vi "Run.vi"(8 "error in (no error)":errorcluster, 10 "Control In":T1={"I-O.lvclass"=refnum, "Gantry"=refnum, "Dispenser"="COM1"}, 11 "Assembly In":refnum<class "Assembly Run.lvclass">) -> (0 "error out":errorcluster, 2 "Control Out":T1={"I-O.lvclass"=refnum, "Gantry"=refnum, "Dispenser"="COM1"}, 3 "Assembly Out":refnum<class "Assembly Run.lvclass">)   [LabVIEW 2018, in "Assembly Run.lvclass"]
uses:
  Assembly Run.lvclass
  Controller/Controllers.ctl
  Controller/I-O/I-O.lvclass
  C:/Program Files (x86)/Aerotech/A3200/LabVIEW/2010/Bin/Aerotech.A3200.dll
  Program Files (x86)/Aerotech/A3200/LabVIEW/2010/Bin/Aerotech.A3200.dll
  Assembly Run.lvclass/Assembly Run.ctl
  Workspace/Fixture.lvclass
  Routine/Routine.lvclass
  Controller/Motion/Motion.lvclass
  Controller/Controller.lvclass
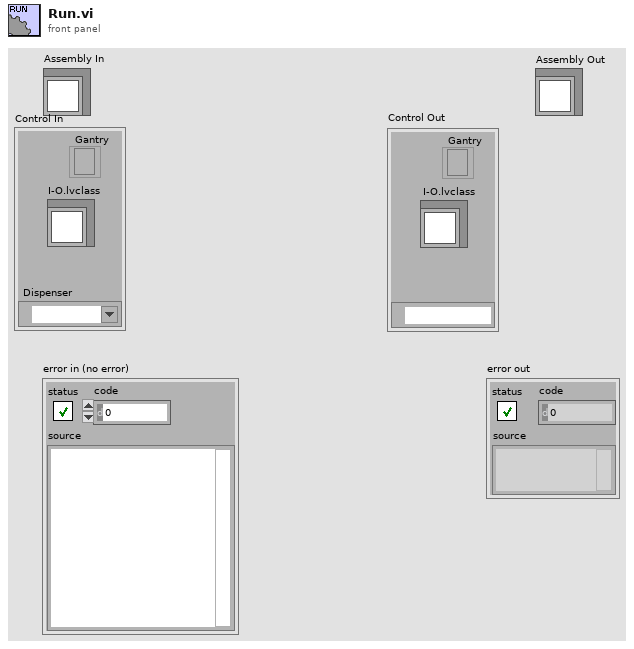
[diagram p1: front panel]
types:
  T1 = typedef "Controller.lvclass/Controllers.ctl" = cluster{"I-O.lvclass":refnum<class "I-O.lvclass">, "Gantry":refnum<k24>, "Dispenser":refnum<visa-resource-name>}
  T2 = typedef "Fixture.lvclass/Workspace.ctl" = cluster{"XYZTheta":dbl[], "Workspace Valve":i32, "Workspace Sensor":i32}
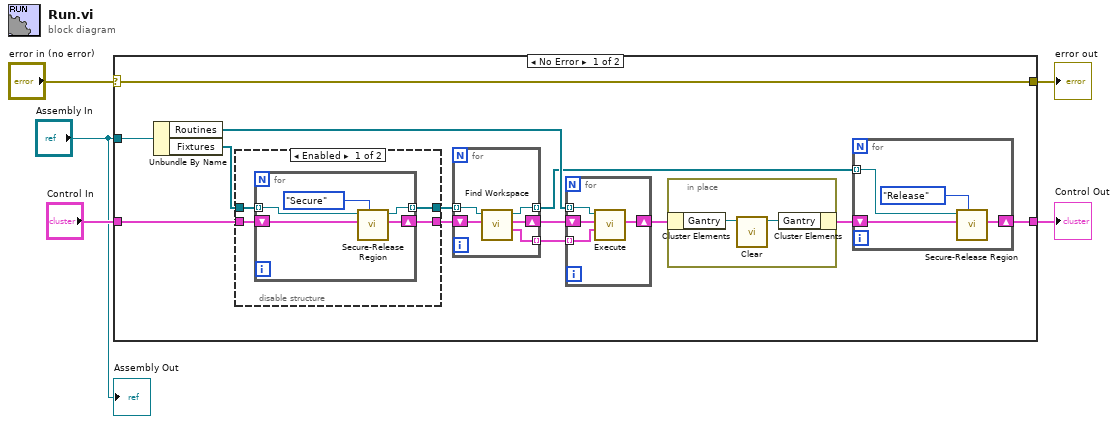
[diagram p0: block diagram]
diagram:
  n1 = case shown="No Error" "error in (no error)" {
    selector: "error in (no error)" -> [w18 w46]
    tunnel: [w18 w46] -> w4
    tunnel: [w12 w45] -> w3
    tunnel: "Assembly In" -> [w10 _]
    tunnel: "Control In" -> [w7 w45]
    frame No Error {
      n2 = Unbundle By Name(w10) -> ("Routines"=w17:refnum<class "Routine.lvclass">[], "Fixtures"=w11:refnum<class "Fixture.lvclass">[])
      n3 = disable-structure shown="Enabled" {
        disable-tunnel: [w22 w29] -> w15
        disable-tunnel: w11 -> [w21 w29]
        disable-tunnel: w7 -> [w20 w28]
        disable-tunnel: [w19 w28] -> w6
        frame Enabled {
          n4 = for {
            tunnel: [w27] -> w22 mode=indexing
            tunnel: w21 -> [w26] mode=indexing
            shift-right: [w24] -> w19
            shift-left: w20 -> [w25]
            n5 = call-dynamic "Secure-Release Region.vi"("Action"=enum16{"Secure", "Release"}."Secure", "Control In"=w25, "Fixture in"=w26) -> ("Control Out"=w24:T1, "Fixture out"=w27:refnum<class "Fixture.lvclass">)  [unwired: 6 in, 1 out]
          }
        }
        frame Disabled {
        }
      }
      n6 = for {
        tunnel: w15 -> [w44] mode=indexing
        tunnel: [w42] -> w16 mode=indexing
        tunnel: [w43] -> w14 mode=indexing
        shift-right: [w40] -> w9
        shift-left: w6 -> [w41]
        n7 = call-dynamic "Find Workspace.vi"("Control In"=w41, "Workspace In"=w44) -> (1:"Workspace Out"=w42:T2, "Control Out"=w40:T1, 3:"Workspace Out"=w43:refnum<class "Fixture.lvclass">)  [unwired: 6 in, 1 out]
      }
      n8 = for {
        tunnel: w17 -> [w39] mode=indexing
        tunnel: w16 -> [w38] mode=indexing
        shift-right: [w36] -> w8
        shift-left: w9 -> [w37]
        n9 = call-dynamic "Execute.vi"("Workspace"=w38, "Control In"=w37, "Routine in"=w39) -> ("Control Out"=w36:T1)  [unwired: 6 in, 2 out]
      }
      n10 = in-place {
        n11 = in-place-cluster #1(w8) -> ("Gantry"=w34:refnum<k24>)
        n12 = call "Clear.vi"("Gantry In"=w34) -> ("Gantry Out"=w35:refnum<k24>)  [unwired: 9 in, 1 out]
        n13 = in-place-cluster #1("Gantry"=w35) -> (w13:T1)
      }
      n14 = for {
        tunnel: w14 -> [w33] mode=indexing
        shift-right: [w32] -> w12
        shift-left: w13 -> [w31]
        n15 = call-dynamic "Secure-Release Region.vi"("Action"=enum16{"Secure", "Release"}."Release", "Control In"=w31, "Fixture in"=w33) -> ("Control Out"=w32:T1)  [unwired: 6 in, 2 out]
      }
    }
    frame Error {
    }
  }
  "error out" <- w4
  "Control Out" <- w3
  "Assembly Out" <- "Assembly In"
